vi "Set_X.vi"(8 "error in (no error)":errorcluster caption="错误输入（无错误）", 10 "X":dbl, 11 "Point输入":refnum<class "Point.lvclass">) -> (0 "error out":errorcluster caption="错误输出", 3 "Point输出":refnum<class "Point.lvclass">)   [LabVIEW 2011, in "Point.lvclass"]
uses:
  Point.lvclass
  Point.lvclass/Point.ctl
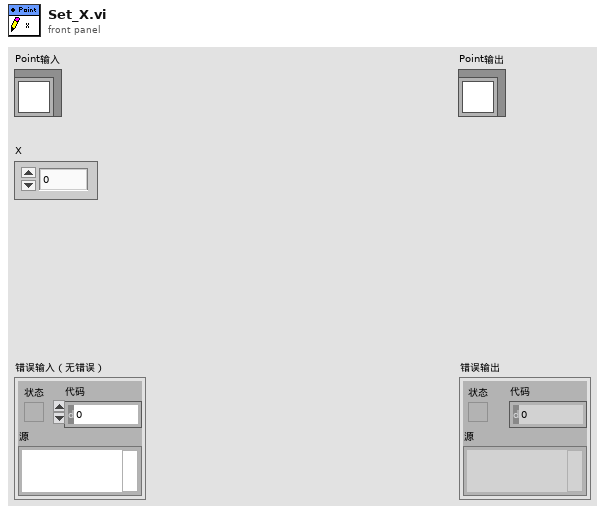
[diagram p1: front panel]
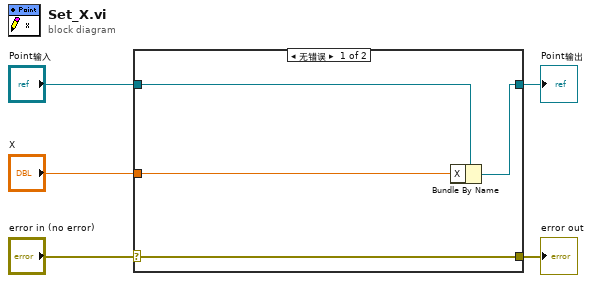
[diagram p0: block diagram]
diagram:
  n1 = case shown="无错误" "error in (no error)" {
    selector: "error in (no error)" -> [w9 w10]
    tunnel: [w9 w10] -> w4
    tunnel: [w7 w11] -> w2
    tunnel: "Point输入" -> [w8 w11]
    tunnel: "X" -> [w6 _]
    frame No Error {
      n2 = Bundle By Name(cluster=w8, "X"=w6) -> (w7:refnum<class "Point.lvclass">)
    }
    frame Error {
    }
  }
  "error out" <- w4
  "Point输出" <- w2
